vi "GDSLvIcon_Convert24bitTo8bitColor.vi"(1 "Color 24bit In":u32(colorbox), 5 "error in (no error)":errorcluster) -> (15 "Adjusted 24bit Color Out":u32(colorbox), 16 "Color out(256)":u8, 17 "Icon 24":i32[][](graph), 19 "error out":errorcluster)   [LabVIEW 2014]
doc: "Converts a 24 bit RGB color to a 8 bit color."
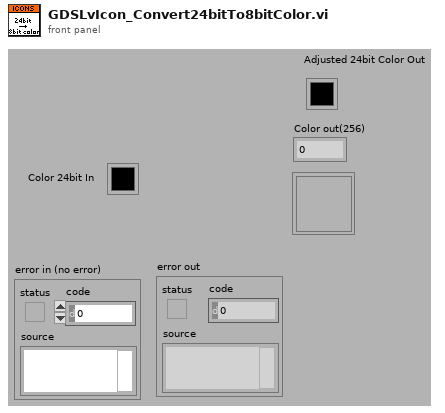
[diagram p1: front panel]
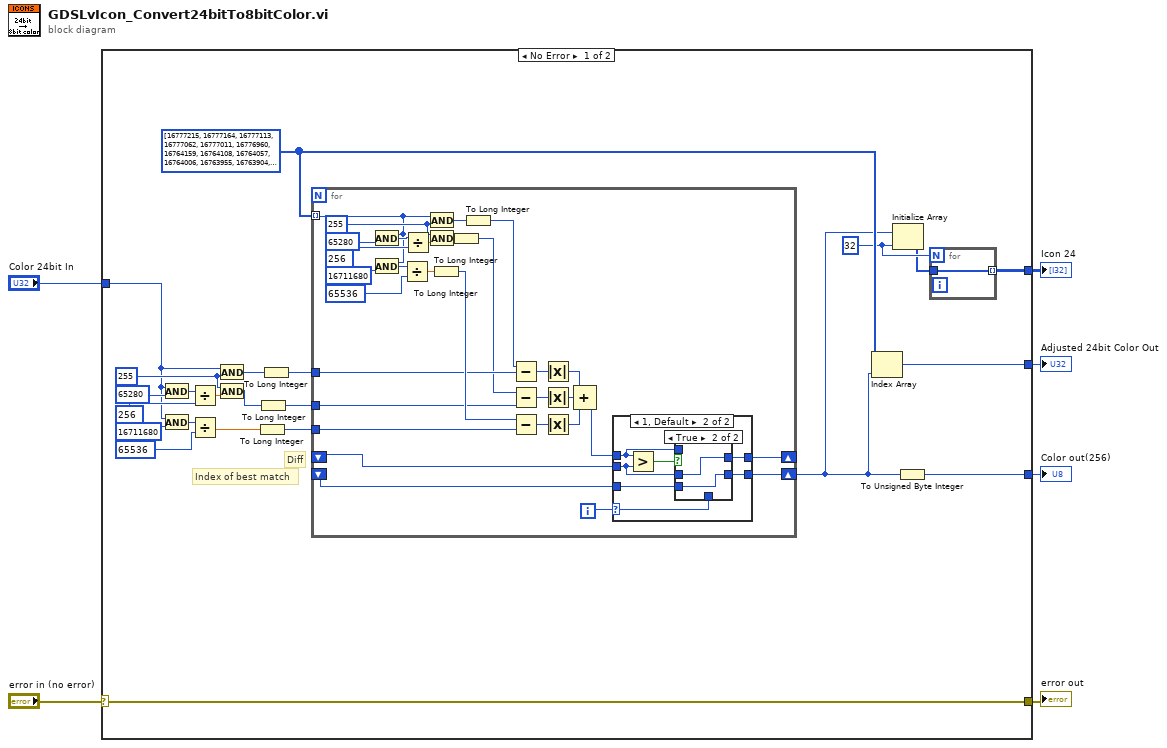
[diagram p0: block diagram]
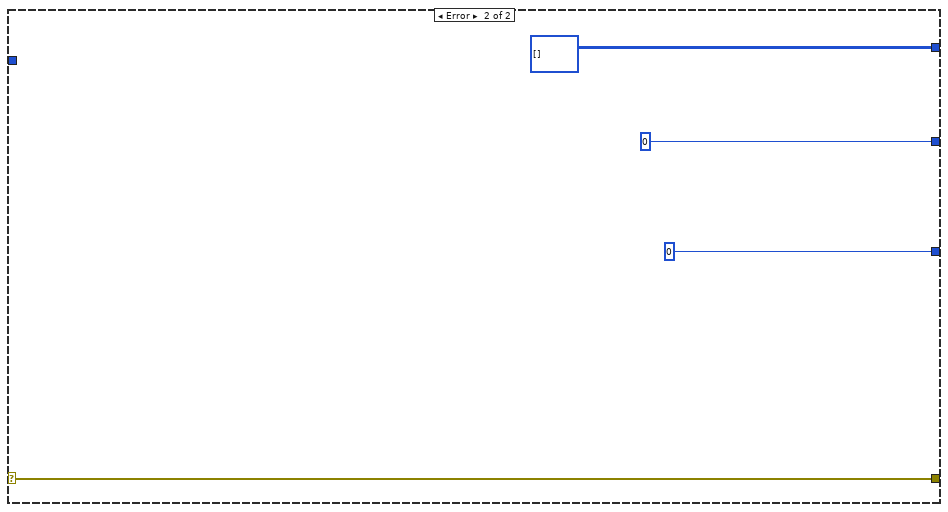
[diagram p4: hidden frame]
diagram:
  n1 = case shown="No Error" "error in (no error)" {
    selector: "error in (no error)" -> [w29 w77]
    tunnel: [w29 w77] -> w5
    tunnel: "Color 24bit In" -> [w10 _]
    tunnel: [w9 i32[][] []] -> w3
    tunnel: [w8 u8 0] -> w2
    tunnel: [w7 u32 0] -> w1
    frame No Error {
      w14 = u32[] [16777215, 16777164, 16777113, 16777062, 16777011, 16776960, 16764159, 16764108, 16764057, 16764006, 16763955, 16763904, 16751103, 16751052, 16751001, 16750950, 16750899, 16750848, 16738047, 16737996, 16737945, 16737894, 16737843, 16737792, 16724991, 16724940, 16724889, 16724838, 16724787, 16724736, 16711935, 16711884, 16711833, 16711782, 16711731, 16711680, 13434879, 13434828, 13434777, 13434726, 13434675, 13434624, 13421823, 13421772, 13421721, 13421670, 13421619, 13421568, 13408767, 13408716, 13408665, 13408614, 13408563, 13408512, 13395711, 13395660, 13395609, 13395558, 13395507, 13395456, 13382655, 13382604, 13382553, 13382502, 13382451, 13382400, 13369599, 13369548, 13369497, 13369446, 13369395, 13369344, 10092543, 10092492, 10092441, 10092390, 10092339, 10092288, 10079487, 10079436, 10079385, 10079334, 10079283, 10079232, 10066431, 10066380, 10066329, 10066278, 10066227, 10066176, 10053375, 10053324, 10053273, 10053222, 10053171, 10053120, 10040319, 10040268, 10040217, 10040166, 10040115, 10040064, 10027263, 10027212, 10027161, 10027110, 10027059, 10027008, 6750207, 6750156, 6750105, 6750054, 6750003, 6749952, 6737151, 6737100, 6737049, 6736998, 6736947, 6736896, 6724095, 6724044, 6723993, 6723942, 6723891, 6723840, 6711039, 6710988, 6710937, 6710886, 6710835, 6710784, 6697983, 6697932, 6697881, 6697830, 6697779, 6697728, 6684927, 6684876, 6684825, 6684774, 6684723, 6684672, 3407871, 3407820, 3407769, 3407718, 3407667, 3407616, 3394815, 3394764, 3394713, 3394662, 3394611, 3394560, 3381759, 3381708, 3381657, 3381606, 3381555, 3381504, 3368703, 3368652, 3368601, 3368550, 3368499, 3368448, 3355647, 3355596, 3355545, 3355494, 3355443, 3355392, 3342591, 3342540, 3342489, 3342438, 3342387, 3342336, 65535, 65484, 65433, 65382, 65331, 65280, 52479, 52428, 52377, 52326, 52275, 52224, 39423, 39372, 39321, 39270, 39219, 39168, 26367, 26316, 26265, 26214, 26163, 26112, 13311, 13260, 13209, 13158, 13107, 13056, 255, 204, 153, 102, 51, 15597568, 14483456, 12255232, 11141120, 8912896, 7798784, 5570560, 4456448, 2228224, 1114112, 60928, 56576, 47872, 43520, 34816, 30464, 21760, 17408, 8704, 4352, 238, 221, 187, 170, 136, 119, 85, 68, 34, 17, 15658734, 14540253, 12303291, 11184810, 8947848, 7829367, 5592405, 4473924, 2236962, 1118481, 0] ("256->24bit colors")
      w13 = 32 ("Dimension Size")
      w21 = u32 255 ("y")
      # "Index of best match"
      # "Diff"
      n2 = And(x=w10, y=u32 65280) -> (x .and. y?=w25:u32)
      n3 = And(x=w10, y=u32 16711680) -> (x .and. y?=w23:u32)
      n4 = Divide(x=w25, y=u32 256) -> (x/y=w22:dbl)
      n5 = Divide(x=w23, y=u32 65536) -> (x/y=w18:dbl)
      n6 = And(x=w10, y=w21) -> (x .and. y?=w20:u32)
      n7 = And(x=w21, y=w22) -> (x .and. y?=w19:i32)
      n8 = To Long Integer(number=w18) -> (32bit integer=w15:i32)
      n9 = To Long Integer(number=w19) -> (32bit integer=w16:i32)
      n10 = To Long Integer(number=w20) -> (32bit integer=w17:i32)
      n11 = for {
        tunnel: w14 -> [w52] mode=indexing
        shift-right: [w39] -> _
        shift-left: _ -> [w38]
        shift-right: [w50] -> w11
        shift-left: _ -> [w37]
        tunnel: w17 -> [w45]
        tunnel: w16 -> [w44]
        tunnel: w15 -> [w43]
        i -> [w51]
        w60 = u32 255 ("y")
        n12 = And(x=w52, y=u32 65280) -> (x .and. y?=w56:u32)
        n13 = And(x=w52, y=u32 16711680) -> (x .and. y?=w58:u32)
        n14 = Divide(x=w58, y=u32 65536) -> (x/y=w47:dbl)
        n15 = Divide(x=w56, y=u32 256) -> (x/y=w59:dbl)
        n16 = And(x=w52, y=w60) -> (x .and. y?=w49:u32)
        n17 = And(x=w60, y=w59) -> (x .and. y?=w48:i32)
        n18 = To Long Integer(number=w47) -> (32bit integer=w46:i32)
        n19 = To Long Integer(number=w48) -> (32bit integer=w41:i32)
        n20 = To Long Integer(number=w49) -> (32bit integer=w42:i32)
        n21 = Subtract(x=w42, y=w45) -> (x-y=w36:i32)
        n22 = Subtract(x=w41, y=w44) -> (x-y=w35:i32)
        n23 = Subtract(x=w46, y=w43) -> (x-y=w34:i32)
        n24 = Absolute Value(x=w36) -> (abs(x)=w33:i32)
        n25 = Absolute Value(x=w35) -> (abs(x)=w32:i32)
        n26 = Absolute Value(x=w34) -> (abs(x)=w31:i32)
        n27 = Compound Arithmetic op=ADD(w33, w32, w31) -> (w40:i32)
        n28 = case shown="1, Default" w51 {
          selector: w51 -> [w62 w63]
          tunnel: [w62 w65] -> w50
          tunnel: w40 -> [w61 w64]
          tunnel: [w61 w67] -> w39
          tunnel: w38 -> [_ w68]
          tunnel: w37 -> [_ w66]
          frame 0 {
          }
          frame 1, Default {
            n29 = Greater?(x=w64, y=w68) -> (0:w69:bool)
            n30 = case shown="True" w69 {
              tunnel: w68 -> [_ w73]
              tunnel: [w71 w73] -> w67
              tunnel: w66 -> [_ w72]
              tunnel: [w70 w72] -> w65
              tunnel: w64 -> [w71 _]
              tunnel: w63 -> [w70 _]
              frame False {
              }
              frame True {
              }
            }
          }
        }
      }
      n31 = Index Array(array=w14, index=w11) -> (element=w7:u32)
      n32 = Initialize Array(w11, w13) -> (w12:i32[])
      n33 = To Unsigned Byte Integer(number=w11) -> (unsigned 8bit integer=w8:u8)
      n34 = for {
        N: w13 -> [_]
        tunnel: [w30] -> w9 mode=indexing
        tunnel: w12 -> [w30]
      }
    }
    frame Error {
    }
  }
  "error out" <- w5
  "Icon 24" <- w3
  "Adjusted 24bit Color Out" <- w1
  "Color out(256)" <- w2
